vi "Read Timer Loop Timeout Period--constant.vi"() -> (3 "Timer":i32)   [LabVIEW 2024, in "IOLink.lvlib"]
uses:
  IOLink.lvlib
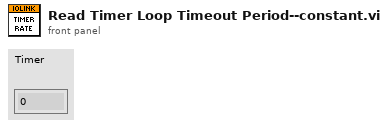
[diagram p1: front panel]
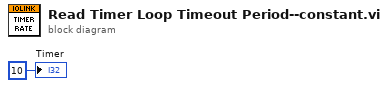
[diagram p0: block diagram]
diagram:
  "Timer" <- 10 ("Timer")
